vi "Realsense Cam Config Cam Options.vi"(8 "error in (no error)":errorcluster, 11 "Realsense Cam in":refnum<class "Realsense Cam.lvclass">) -> (0 "error out":errorcluster, 3 "Realsense Cam out":refnum<class "Realsense Cam.lvclass">)   [LabVIEW 2018, in "Realsense Cam.lvclass"]
uses:
  Realsense Cam.lvclass
  Realsense Cam.lvclass/Realsense Cam.ctl
  Temp/realsense_labview_sdk/RealSense SDK2.11.0 for LabVIEW/libRealSense3.lvlib
panel:
  out "Set Option error":string
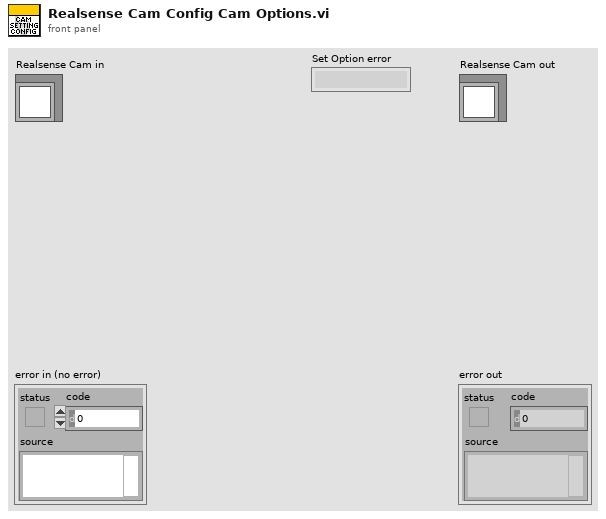
[diagram p1: front panel]
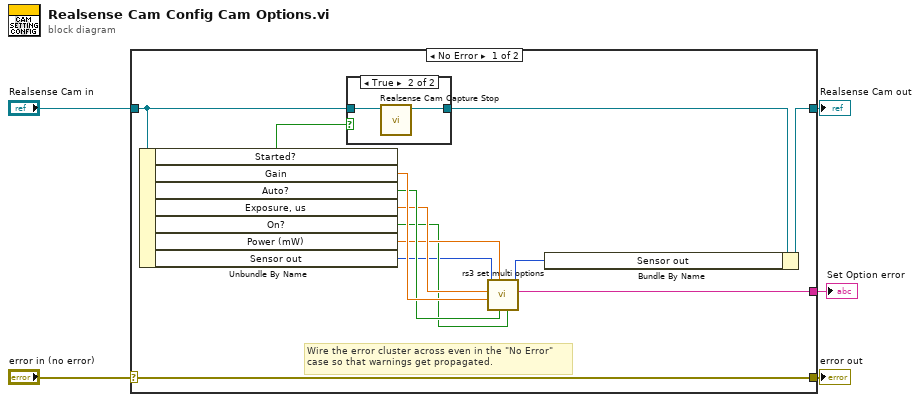
[diagram p0: block diagram]
diagram:
  n1 = case shown="No Error" "error in (no error)" {
    selector: "error in (no error)" -> [w18 w23]
    tunnel: [w18 w23] -> w4
    tunnel: [w7 w22] -> w2
    tunnel: "Realsense Cam in" -> [w16 w22]
    tunnel: [w6 _] -> w1
    frame No Error {
      # "Wire the error cluster across even in the \"No Error\"\ncase so that warnings get propagated."
      n2 = Unbundle By Name(w16) -> ("Started?"=w17:bool, "Gain"=w15:sgl, "Auto?"=w14:bool, "Exposure, us"=w13:sgl, "On?"=w11:bool, "Power (mW)"=w12:dbl, "Sensor out"=w10:u64)
      n3 = case shown="True" w17 {
        tunnel: w16 -> [w19 w21]
        tunnel: [w19 w20] -> w9
        frame False {
        }
        frame True {
          n4 = call-dynamic "Realsense Cam Capture Stop.vi"("Realsense Cam in"=w21) -> ("Realsense Cam out"=w20:refnum<class "Realsense Cam.lvclass">)  [unwired: 8 in, 2 out]
        }
      }
      n5 = call "rs3 set multi options.vi"("laser on/off"=w11, "autoexposure"=w14, "Laser power, mW (0-360)"=w12, "Gain(16-248)"=w15, "Exposure, us"=w13, "Sensor in"=w10) -> ("Set Option error"=w6:string, "Sensor out"=w8:u64)  [unwired: 3 in, 1 out]
      n6 = Bundle By Name(cluster=w9, "Sensor out"=w8) -> (w7:refnum<class "Realsense Cam.lvclass">)
    }
    frame Error {
    }
  }
  "error out" <- w4
  "Realsense Cam out" <- w2
  "Set Option error" <- w1
